vi "Format List Data.vi"(7 "Include All time":bool, 10 "#Offset":i32, 11 "Data":T1[](array[typedef]) {"Direction" items=["Tx", "Rx"]; "CANType" items=["CAN", "CANFD", "CANFD加速"]}) -> (3 "List Data":string[][](array[string]))   [LabVIEW 2011, in "CAN FD.lvlib"]
uses:
  CAN FD.lvlib
  Typedef/CAN Data.ctl
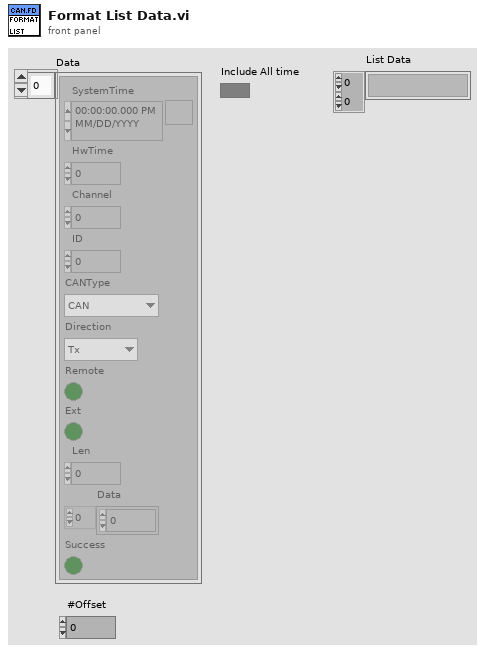
[diagram p1: front panel]
types:
  T1 = typedef "CAN FD.lvlib/CAN Data.ctl" = cluster{"SystemTime":timestamp, "HwTime":dbl, "Channel":u8, "ID":u32, "CANType":i16, "Direction":i16, "Remote":bool, "Ext":bool, "Len":u8, "Data":u8[], "Success":bool}
  T2 = enum16{"#", "TimeStamp", "Channel", "ID", "Type", "Format", "CANtype", "Dir", "Len", "Data", "HwTime", "SysTime"}[]
  T3 = typedef "CAN FD.lvlib/Config.ctl" = cluster{"TimeFormat":u16, "ID Format":u16, "Data Format":u16, "ListLen":u32}
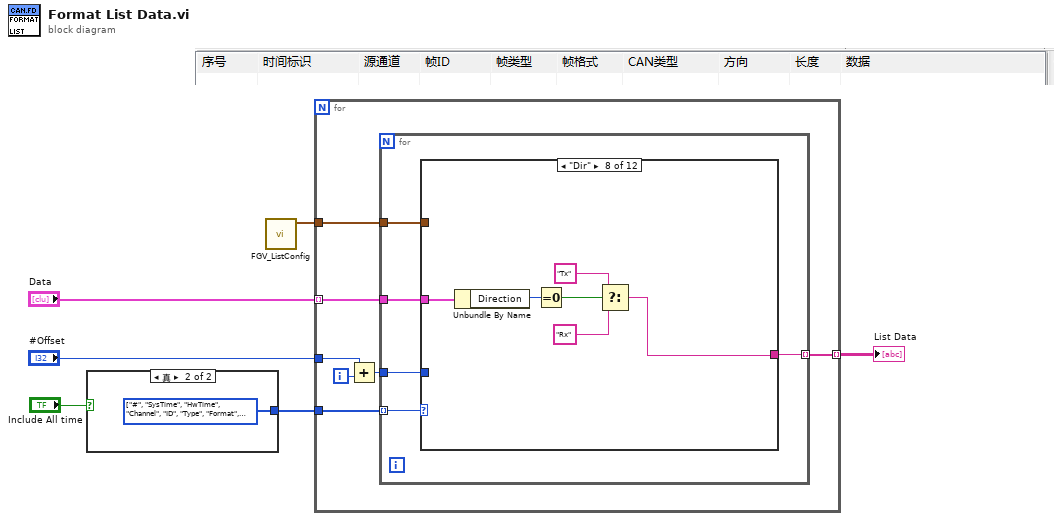
[diagram p0: block diagram]
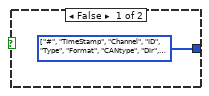
[diagram p2: hidden frame]
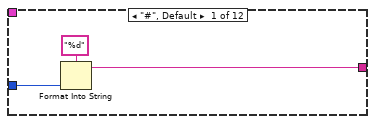
[diagram p3: hidden frame]
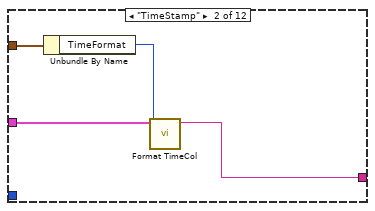
[diagram p4: hidden frame]
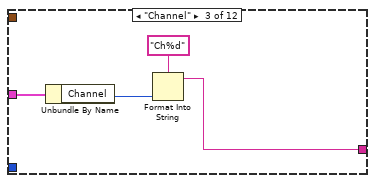
[diagram p5: hidden frame]
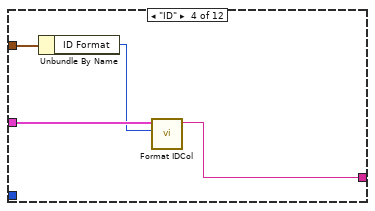
[diagram p6: hidden frame]
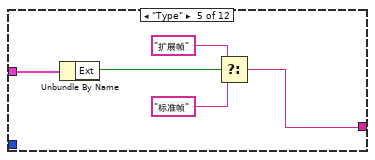
[diagram p7: hidden frame]
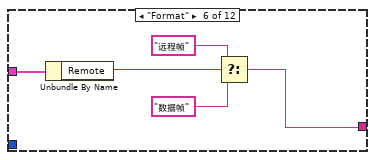
[diagram p8: hidden frame]
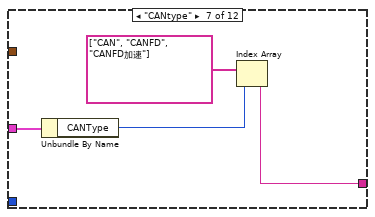
[diagram p9: hidden frame]
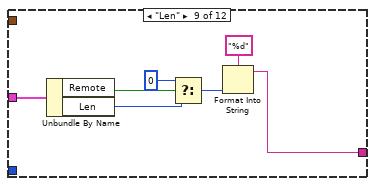
[diagram p10: hidden frame]
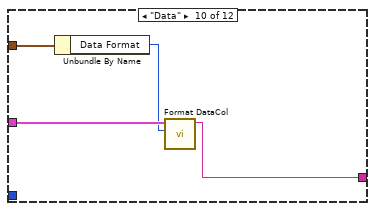
[diagram p11: hidden frame]
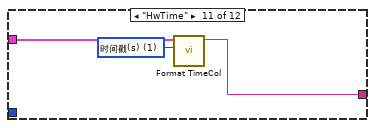
[diagram p12: hidden frame]
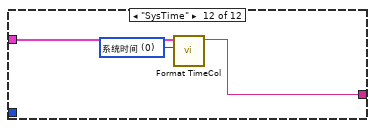
[diagram p13: hidden frame]
diagram:
  n1 = case shown="真" "Include All time" {
    tunnel: [w7 w8] -> w1
    frame False {
      w7 = T2 [enum."#", enum."TimeStamp", enum."Channel", enum."ID", enum."Type", enum."Format", enum."CANtype", enum."Dir", enum."Len", enum."Data"] items=["#", "TimeStamp", "Channel", "ID", "Type", "Format", "CANtype", "Dir", "Len", "Data", "HwTime", "SysTime"]
    }
    frame True {
      w8 = T2 [enum."#", enum."SysTime", enum."HwTime", enum."Channel", enum."ID", enum."Type", enum."Format", enum."CANtype", enum."Dir", enum."Len", enum."Data"] items=["#", "TimeStamp", "Channel", "ID", "Type", "Format", "CANtype", "Dir", "Len", "Data", "HwTime", "SysTime"]
    }
  }
  n2 = call "FGV_ListConfig.vi"() -> ("Config out"=w6:T3)  [unwired: 10 in, 1 out]
  n3 = for {
    tunnel: "Data" -> [w15] mode=indexing
    tunnel: w6 -> [w10]
    tunnel: "#Offset" -> [w13]
    tunnel: [w11] -> w5 mode=indexing
    tunnel: w1 -> [w9]
    i -> [w14]
    n4 = Add(x=w13, y=w14) -> (x+y=w12:i32)
    n5 = for {
      tunnel: w15 -> [w18]
      tunnel: w12 -> [w20]
      tunnel: [w19] -> w11 mode=indexing
      tunnel: w10 -> [w17]
      tunnel: w9 -> [w16] mode=indexing
      n6 = case shown="\"Dir\"" w16 {
        tunnel: w20 -> [w23 _ _ _ _ _ _ _ _ _ _ _]
        tunnel: [w21 w24 w28 w32 w36 w41 w46 w51 w57 w63 w67 w70] -> w19
        tunnel: w18 -> [_ w26 w31 w34 w40 w45 w49 w55 w62 w65 w69 w72]
        tunnel: w17 -> [_ w27 _ w35 _ _ _ _ _ w66 _ _]
        frame "#", Default {
          n7 = Format Into String(format string="%d" ("格式字符串"), w23) -> (resulting string=w21:string)  [unwired: 2 in, 1 out]
        }
        frame "TimeStamp" {
          n8 = Unbundle By Name(w27) -> ("TimeFormat"=w25:u16)
          n9 = call "Format TimeCol.vi"("TimeFormat"=w25, "Data"=w26) -> ("Time str"=w24:string)  [unwired: 9 in]
        }
        frame "Channel" {
          n10 = Unbundle By Name(w31) -> ("Channel"=w30:u8)
          n11 = Format Into String(format string="Ch%d" ("格式字符串"), w30) -> (resulting string=w28:string)  [unwired: 2 in, 1 out]
        }
        frame "ID" {
          n12 = Unbundle By Name(w35) -> ("ID Format"=w33:u16)
          n13 = call "Format IDCol.vi"("ID Format"=w33, "Data"=w34) -> ("ID str"=w32:string)  [unwired: 9 in]
        }
        frame "Type" {
          n14 = Unbundle By Name(w40) -> ("Ext"=w39:bool)
          n15 = Select(t="扩展帧" ("格式字符串"), s=w39, f="标准帧" ("格式字符串")) -> (s? t:f=w36:string)
        }
        frame "Format" {
          n16 = Unbundle By Name(w45) -> ("Remote"=w44:bool)
          n17 = Select(t="远程帧" ("格式字符串"), s=w44, f="数据帧" ("格式字符串")) -> (s? t:f=w41:string)
        }
        frame "CANtype" {
          n18 = Unbundle By Name(w49) -> ("CANType"=w47:i16)
          n19 = Index Array(array=string[] ["CAN", "CANFD", "CANFD加速"], index=w47) -> (element=w46:string)
        }
        frame "Dir" {
          n20 = Unbundle By Name(w55) -> ("Direction"=w54:i16)
          n21 = Equal To 0?(x=w54) -> (x = 0?=w50:bool)
          n22 = Select(t="Tx" ("格式字符串"), s=w50, f="Rx" ("格式字符串")) -> (s? t:f=w51:string)
        }
        frame "Len" {
          n23 = Unbundle By Name(w62) -> ("Remote"=w61:bool, "Len"=w60:u8)
          n24 = Select(t=u8 0, s=w61, f=w60) -> (s? t:f=w58:u8)
          n25 = Format Into String(format string="%d" ("格式字符串"), w58) -> (resulting string=w57:string)  [unwired: 2 in, 1 out]
        }
        frame "Data" {
          n26 = Unbundle By Name(w66) -> ("Data Format"=w64:u16)
          n27 = call "Format DataCol.vi"("Data Format"=w64, "Data"=w65) -> ("ID str"=w63:string)  [unwired: 9 in]
        }
        frame "HwTime" {
          w68 = u16 1 items=["系统时间", "时间戳(s)"] ("TimeFormat")
          n28 = call "Format TimeCol.vi"("TimeFormat"=w68, "Data"=w69) -> ("Time str"=w67:string)  [unwired: 9 in]
        }
        frame "SysTime" {
          w71 = u16 0 items=["系统时间", "时间戳(s)"] ("TimeFormat")
          n29 = call "Format TimeCol.vi"("TimeFormat"=w71, "Data"=w72) -> ("Time str"=w70:string)  [unwired: 9 in]
        }
      }
    }
  }
  "List Data" <- w5
